vi "test Fix Relocated Modules Updates Connections.vi"(8 "error in (no error)":errorcluster, 11 "TestCase in":refnum<class "Routing and Faulting Scripting Unit Tests.lvclass">) -> (0 "error out":errorcluster, 3 "TestCase out":refnum<class "Routing and Faulting Scripting Unit Tests.lvclass">)   [LabVIEW 2017, in "Routing and Faulting Scripting Unit Tests.lvclass"]
uses:
  Routing and Faulting Scripting Unit Tests.lvclass
  Shared/VeriStand SLSC Scripting/Controls/SLSC Chassis ID.ctl
  Shared/Channel States.ctl
  Shared/Routing State.ctl
  Shared/Connection.ctl
  Routing and Faulting Scripting Unit Tests.lvclass/Routing and Faulting Scripting Unit Tests.ctl
  NationalInstruments.VeriStand.SystemDefinitionAPI
  <vilib>/addons/_JKI Toolkits/VI Tester/TestCase.llb/TestCase.lvclass
  Routing and Faulting Scripting.lvlib
  Fake Hardware Custom Device/Fake Hardware Custom Device.lvlib
  Shared/VeriStand SLSC Scripting/VeriStand SLSC Scripting.lvlib
  Shared/Routing and Faulting Hardware API/Routing and Faulting Hardware API.lvlib
  Shared/Routing and Faulting Shared.lvlib
  C:/Program Files (x86)/National Instruments/LabVIEW 2017/vi.lib/addons/_JKI Toolkits/VI Tester/TestCase.llb/TestCase.lvclass
panel:
  in  "Save?":bool
  out "Output Filename":string
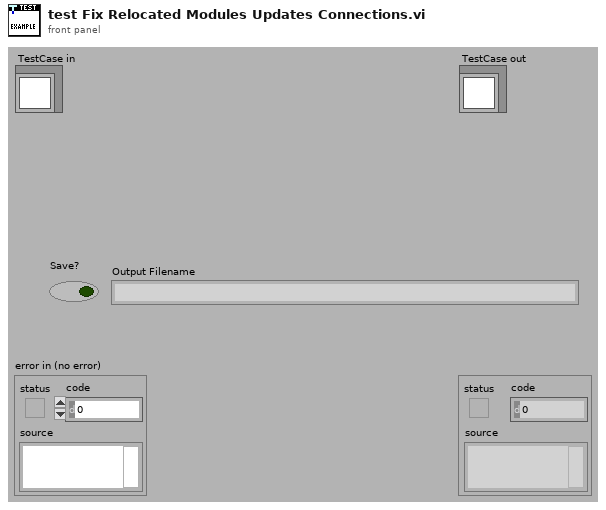
[diagram p1: front panel]
types:
  T1 = typedef "Routing and Faulting Shared.lvlib/Channel States.ctl" = T2[]
  T2 = typedef "Routing and Faulting Shared.lvlib/Routing State.ctl" = cluster{"Name":string, "Description":string, "Value":i32, "Connection List":T3[]}
  T3 = typedef "Routing and Faulting Shared.lvlib/Connection.ctl" = cluster{"Module":string, "Source":string, "Destination":string}
  T4 = typedef "VeriStand SLSC Scripting.lvlib/SLSC Chassis ID.ctl" = cluster{"Name or IP":string, "ChassisIDType":i32, "chassisType":i32}
  T5 = typedef "Custom Device API.lvlib/Custom Device Item Ref.ctl" = u64
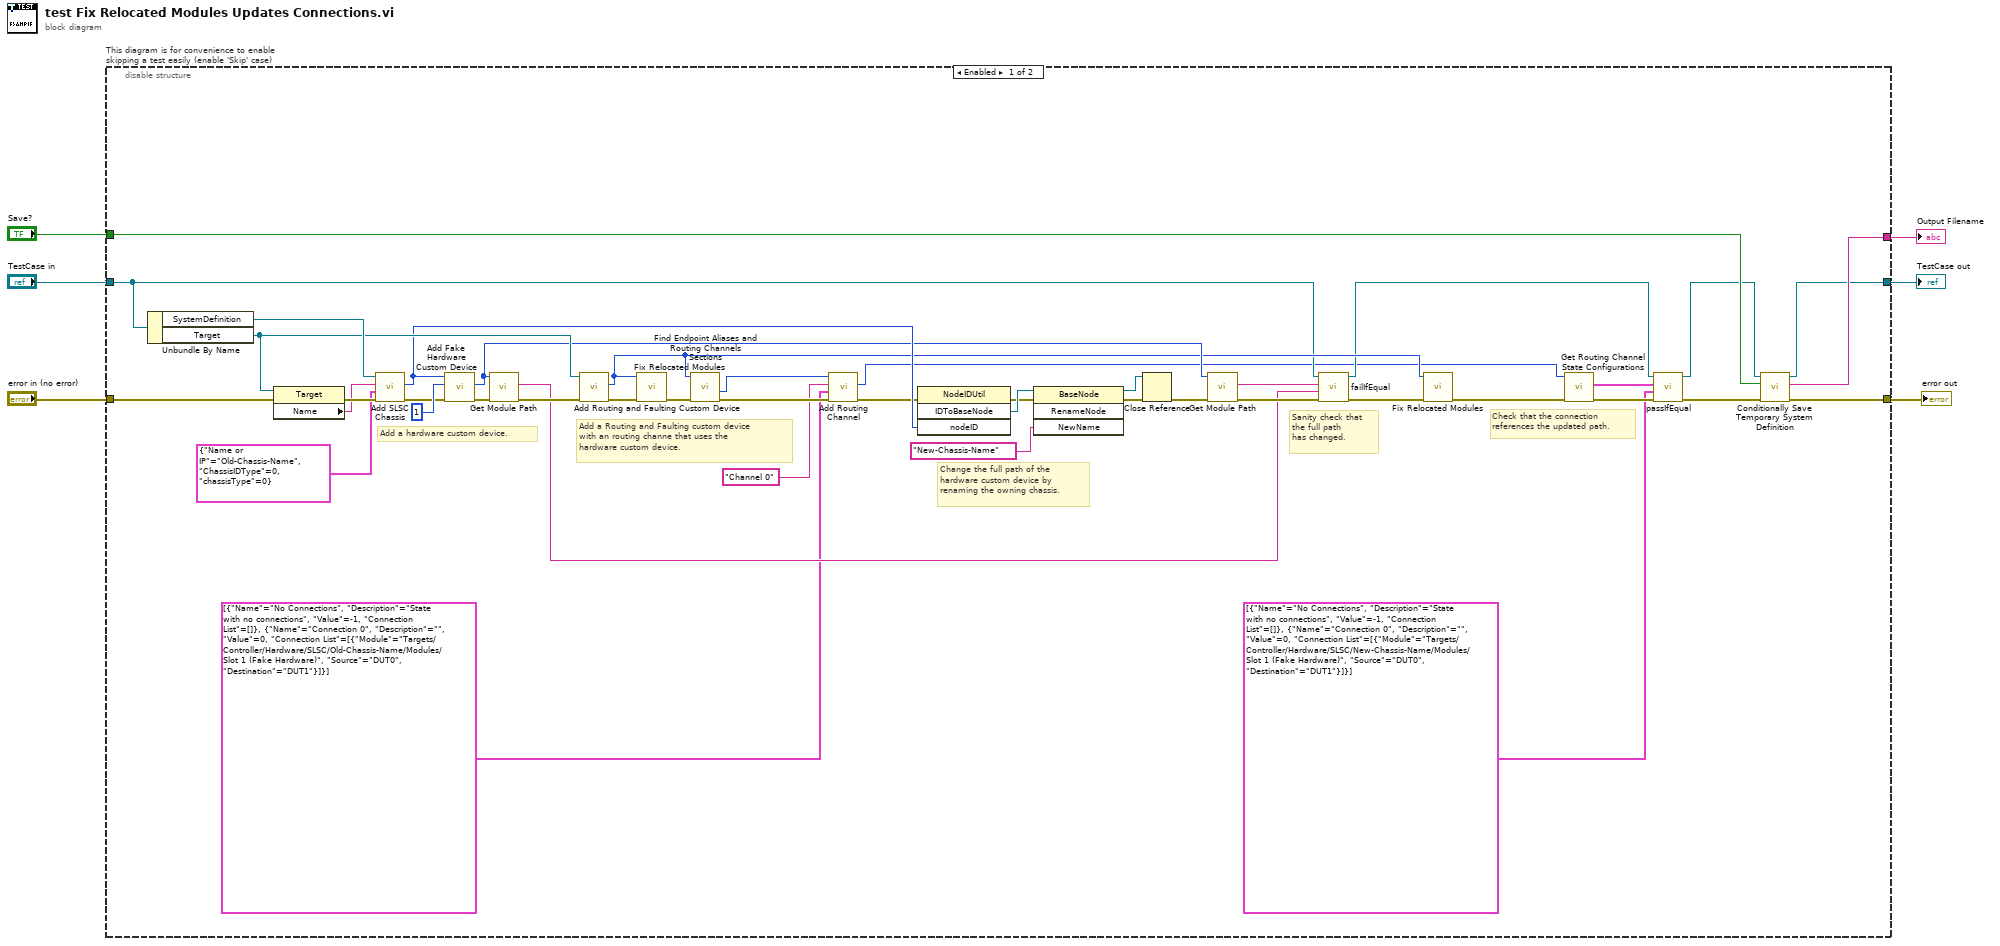
[diagram p0: block diagram]
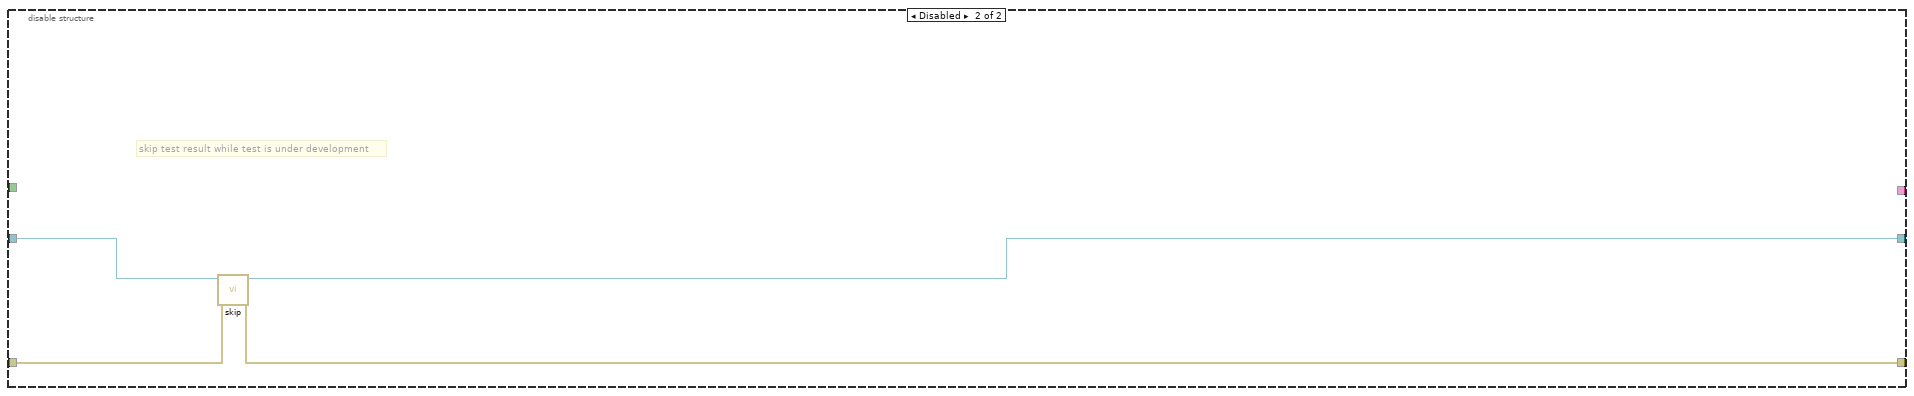
[diagram p2: hidden frame]
diagram:
  n1 = disable-structure "This diagram is for convenience to enable skipping a test easily (enable 'Skip' case)" shown="Enabled" {
    disable-tunnel: "TestCase in" -> [w17 w53]
    disable-tunnel: [w47 w51] -> w3
    disable-tunnel: [w48 w52] -> w5
    disable-tunnel: "error in (no error)" -> [w44 w50]
    disable-tunnel: [w49 _] -> w2
    disable-tunnel: "Save?" -> [w46 _]
    frame Enabled {
      # "Check that the connection\nreferences the updated path."
      # "Sanity check that\nthe full path\nhas changed."
      # "Change the full path of the\nhardware custom device by\nrenaming the owning chassis."
      # "Add a Routing and Faulting custom device\nwith an routing channe that uses the\nhardware custom device."
      # "Add a hardware custom device."
      n2 = Unbundle By Name(w17) -> ("SystemDefinition"=w45:refnum<k24>, "Target"=w39:refnum<k24>)
      n3 = property class="Target"(reference=w39, error in=w44) -> (error out=w43:errorcluster, "Name"=w41:string)  [unwired: 1 out]
      n4 = call "Add SLSC Chassis.vi"("error in (no error)"=w43, "SLSC Chassis ID"=T4 {"Name or IP"="Old-Chassis-Name", "ChassisIDType"=0, "chassisType"=0}, "Target Name"=w41, "SysDef in"=w45) -> ("error out"=w34:errorcluster, "SLSC Chassis"=w27:u64)  [unwired: 5 in, 1 out]
      n5 = call "Add Fake Hardware Custom Device.vi"("error in (no error)"=w34, "Slot Number"=1, "SLSC Chassis Ref"=w27) -> ("error out"=w29:errorcluster, "Fake Hardware Custom Device Ref"=w25:T5)  [unwired: 6 in, 1 out]
      n6 = call "Get Module Path.vi"("error in (no error)"=w29, "Hardware Ref in"=w25) -> ("error out"=w28:errorcluster, "Resource"=w21:string)  [unwired: 6 in, 2 out]
      n7 = call "Add Routing and Faulting Custom Device.vi"("error in (no error)"=w28, "Target in"=w39) -> ("error out"=w38:errorcluster, "Routing and Faulting Custom Device Ref"=w19:T5)  [unwired: 7 in, 1 out]
      n8 = call "Fix Relocated Modules.vi"("error in (no error)"=w38, "Routing and Faulting Ref in"=w19) -> ("error out"=w31:errorcluster)  [unwired: 8 in, 1 out]
      n9 = call "Find Endpoint Aliases and Routing Channels Sections.vi"("error in (no error)"=w31, "Routing and Faulting Custom Device Ref in"=w19) -> ("error out"=w30:errorcluster, "Routing Channels Ref"=w12:T5)  [unwired: 6 in, 2 out]
      n10 = call "Add Routing Channel.vi"("error in (no error)"=w30, "State Configurations"=T1 [{"Name"="No Connections", "Description"="State with no connections", "Value"=-1, "Connection List"=[]}, {"Name"="Connection 0", "Description"="", "Value"=0, "Connection List"=[{"Module"="Targets/Controller/Hardware/SLSC/Old-Chassis-Name/Modules/Slot 1 (Fake Hardware)", "Source"="DUT0", "Destination"="DUT1"}]}], "Channel Name"="Channel 0" ("Alias"), "Routing Channels Ref in"=w12) -> ("error out"=w26:errorcluster, "Channel Ref"=w8:T5)  [unwired: 5 in, 1 out]
      n11 = invoke class="NodeIDUtil" method="IDToBaseNode"(error in=w26, "nodeID"=w27) -> (error out=w35:errorcluster, "IDToBaseNode"=w37:refnum<k24>)  [unwired: 2 in, 2 out]
      n12 = invoke class="BaseNode" method="RenameNode"(reference=w37, error in=w35, "NewName"="New-Chassis-Name") -> (reference out=w32:refnum<k24>, error out=w33:errorcluster)  [unwired: 1 in, 2 out]
      n13 = Close Reference(reference=w32, error in (no error)=w33) -> (error out=w24:errorcluster)
      n14 = call "Get Module Path.vi"("error in (no error)"=w24, "Hardware Ref in"=w25) -> ("error out"=w23:errorcluster, "Resource"=w22:string)  [unwired: 6 in, 2 out]
      n15 = call-dynamic "failIfEqual.vi"("error in (no error)"=w23, "y"=w21, "x"=w22, "TestCase in"=w17) -> ("error out"=w20:errorcluster, "TestCase out"=w16:refnum<class "Routing and Faulting Scripting Unit Tests.lvclass">)  [unwired: 6 in]
      n16 = call "Fix Relocated Modules.vi"("error in (no error)"=w20, "Routing and Faulting Ref in"=w19) -> ("error out"=w7:errorcluster)  [unwired: 8 in, 1 out]
      n17 = call "Get Routing Channel State Configurations.vi"("error in (no error)"=w7, "Channel Ref in"=w8) -> ("error out"=w10:errorcluster, "State Configurations"=w11:T1)  [unwired: 7 in, 1 out]
      n18 = call-dynamic "passIfEqual.vi"("error in (no error)"=w10, "y"=T1 [{"Name"="No Connections", "Description"="State with no connections", "Value"=-1, "Connection List"=[]}, {"Name"="Connection 0", "Description"="", "Value"=0, "Connection List"=[{"Module"="Targets/Controller/Hardware/SLSC/New-Chassis-Name/Modules/Slot 1 (Fake Hardware)", "Source"="DUT0", "Destination"="DUT1"}]}] ("State Configurations"), "x"=w11, "TestCase in"=w16) -> ("error out"=w14:errorcluster, "TestCase out"=w15:refnum<class "Routing and Faulting Scripting Unit Tests.lvclass">)  [unwired: 6 in]
      n19 = call "Conditionally Save Temporary System Definition.vi"("error in (no error)"=w14, "Save?"=w46, "Test Case"=w15) -> ("error out"=w48:errorcluster, "filename"=w49:string, "Test Case"=w47:refnum<class "Routing and Faulting Scripting Unit Tests.lvclass">)  [unwired: 6 in]
    }
    frame Disabled {
      # "skip test result while test is under development"
      n20 = call <vilib>:"skip.vi"("error in (no error)"=w50, "TestCase in"=w53) -> ("error out"=w52:errorcluster, "TestCase out"=w51:refnum<class "Routing and Faulting Scripting Unit Tests.lvclass">)  [unwired: 8 in]
    }
  }
  "error out" <- w5
  "TestCase out" <- w3
  "Output Filename" <- w2
